vi "Close.vi"(8 "error in (no error)":errorcluster, 11 "QPA Measurement in":refnum<class "QPA Measurement.lvclass">) -> (0 "error out":errorcluster, 3 "QPA Measurement out":refnum<class "QPA Measurement.lvclass">)   [LabVIEW 2016, in "QPA Measurement.lvlib" / "QPA Measurement.lvclass"]
uses:
  QPA Measurement.lvclass
  QPA Measurement.lvclass/QPA Measurement.ctl
  Protected Methods/Read Default Steps Database.vi
  Protected Methods/Read Dut Setup Step.vi
  Protected Methods/Read RF Waveform Database.vi
  Protected Methods/Read External Network Step.vi
  Plugins/Measurement Interface.lvlibp/Measurement Interface.lvclass
  Waveform Manager/QPA MSMT Waveform Manager.lvclass
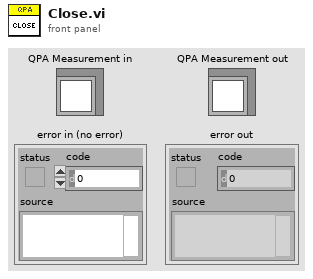
[diagram p1: front panel]
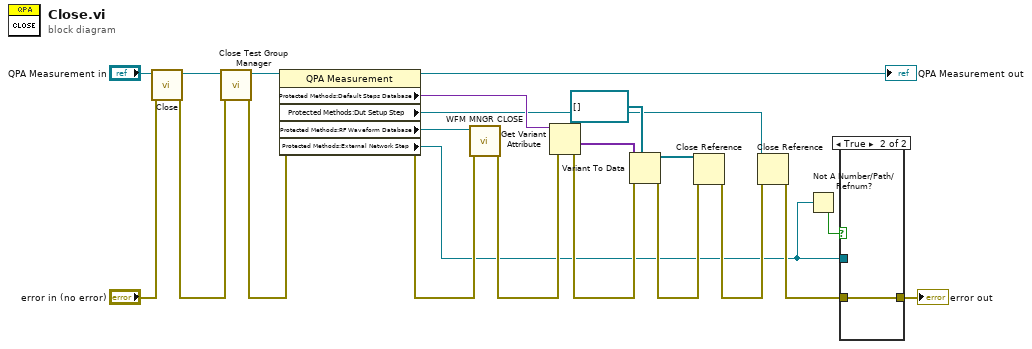
[diagram p0: block diagram]
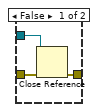
[diagram p2: hidden frame]
diagram:
  n1 = call-parent "Close.vi"("error in (no error)"="error in (no error)", "Measurement Interface in"="QPA Measurement in") -> ("error out"=w22:errorcluster, "Measurement Interface out"=w2:refnum<class "QPA Measurement.lvclass">)  [unwired: 8 in]
  n2 = call "Close Test Group Manager.vi"("error in (no error)"=w22, "QPA Measurement in"=w2) -> ("error out"=w3:errorcluster, "QPA Measurement out"=w1:refnum<class "QPA Measurement.lvclass">)  [unwired: 8 in]
  n3 = property class="QPA Measurement"(reference=w1, error in=w3) -> (reference out=→"QPA Measurement out":refnum<class "QPA Measurement.lvclass">, error out=w9:errorcluster, "Protected Methods:Default Steps Database"=w18:variant, "Protected Methods:Dut Setup Step"=w10:refnum<k7>, "Protected Methods:RF Waveform Database"=w7:refnum<class "QPA MSMT Waveform Manager.lvclass">, "Protected Methods:External Network Step"=w5:refnum<k7>)
  n4 = call "WFM MNGR CLOSE.vi"("error in (no error)"=w9, "WFM MNGR in"=w7) -> ("error out"=w8:errorcluster)  [unwired: 8 in, 1 out]
  n5 = Get Variant Attribute(Variant=w18, error in=w8) -> (values=w17:variant[], error out=w15:errorcluster)  [unwired: 2 in, 2 out]
  n6 = Variant To Data(error in=w15, type=refnum<k7>[] [], Variant=w17) -> (data=w14:refnum<k7>[], error out=w13:errorcluster)
  n7 = Close Reference(reference=w14, error in (no error)=w13) -> (error out=w12:errorcluster)
  n8 = Close Reference(reference=w10, error in (no error)=w12) -> (error out=w11:errorcluster)
  n9 = Not A Number/Path/Refnum?(number/path/refnum=w5) -> (NaN/Path/Refnum?=w4:bool)
  n10 = case shown="True" w4 {
    tunnel: w11 -> [w25 w26]
    tunnel: [w24 w26] -> w6
    tunnel: w5 -> [w23 _]
    frame False {
      n11 = Close Reference(reference=w23, error in (no error)=w25) -> (error out=w24:errorcluster)
    }
    frame True {
    }
  }
  "error out" <- w6
